vi "test subVI - Caraya.vi"(8 "error in (no error)":errorcluster, 11 "Report Path":path) -> (0 "error out":errorcluster)   [LabVIEW 2020]
uses:
  <vilib>/addons/_JKI Toolkits/Caraya/classes/Test Suite/Define Test Suite (JUnit Report).vi
  <vilib>/addons/_JKI Toolkits/Caraya/classes/Assert/Assert Equal Value and Type_Variant.vi
  <vilib>/addons/_JKI Toolkits/Caraya/classes/Test Suite/Test Suite.lvclass
  <vilib>/addons/_JKI Toolkits/Caraya/classes/Test/Test.lvclass
  <vilib>/addons/_JKI Toolkits/Caraya/classes/Assert/Assert.lvclass
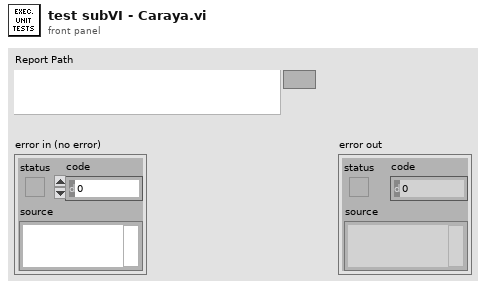
[diagram p1: front panel]
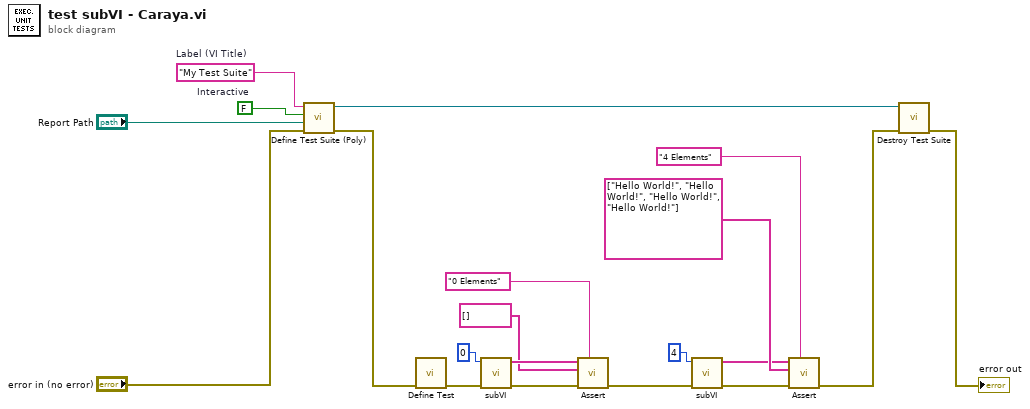
[diagram p0: block diagram]
diagram:
  w3 = "My Test Suite"  # Label (VI Title)
  w4 = FALSE  # Interactive
  n1 = call-poly <vilib>:"Define Test Suite (Poly).vi"("error in (no error)"="error in (no error)", "Report Path"="Report Path", "Interactive"=w4, "Label (VI Title)"=w3) -> ("error out"=w6:errorcluster, "Test Suite"=w5:refnum<class "Test Suite.lvclass">)  [unwired: 6 in]
  n2 = call <vilib>:"Define Test.vi"("error in (no error)"=w6) -> ("error out"=w20:errorcluster)  [unwired: 10 in]
  n3 = call "subVI.vi"("error in (no error)"=w20, "Hello Count"=u32 0) -> ("error out"=w19:errorcluster, "Array of Hello Worlds"=w17:string[])  [unwired: 8 in]
  n4 = call-poly <vilib>:"Assert.vi"("Label"="0 Elements", "error in (no error)"=w19, "Y"=string[] [], "X"=w17) -> ("error out"=w9:errorcluster)  [unwired: 7 in]
  n5 = call "subVI.vi"("error in (no error)"=w9, "Hello Count"=u32 4) -> ("error out"=w10:errorcluster, "Array of Hello Worlds"=w12:string[])  [unwired: 8 in]
  n6 = call-poly <vilib>:"Assert.vi"("Label"="4 Elements", "error in (no error)"=w10, "Y"=string[] ["Hello World!", "Hello World!", "Hello World!", "Hello World!"], "X"=w12) -> ("error out"=w8:errorcluster)  [unwired: 7 in]
  n7 = call-dynamic "Destroy Test Suite.vi"("error in (no error)"=w8, "Test Suite in"=w5) -> ("error out"=→"error out":errorcluster)  [unwired: 9 in]
